vi "add.vi"(10 "x":dbl, 11 "y":dbl) -> (2 "x_y":dbl, 3 "x+y":dbl)   [LabVIEW 2019, in "GettingStarted_5775_Host.lvlib"]
uses:
  GettingStarted_5775_Host.lvlib
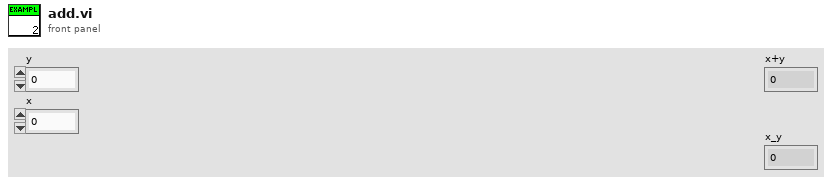
[diagram p1: front panel]
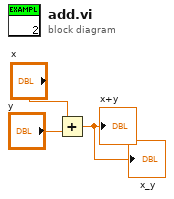
[diagram p0: block diagram]
diagram:
  n1 = Add(x="x", y="y") -> (x+y=→"x+y" →"x_y":dbl)
